vi "FieldInterference.vi"(0 "XCorner":dbl[](array[numeric]), 2 "Rotation":dbl, 5 "YCorner":dbl[](array[numeric]), 9 "Xsonde":dbl, 11 "Ysonde":dbl, 13 "Direction":dbl) -> (3 "vxx":dbl, 6 "XCible":dbl, 10 "YCible":dbl, 14 "vyy":dbl)   [LabVIEW 2011]
panel:
  out "D":bool
  out "C":bool
  out "A":bool
  out "B":bool
  out "d1y":dbl
  out "d1x":dbl
  out "c1y":dbl
  out "c1x":dbl
  out "b1y":dbl
  out "b1x":dbl
  out "output variable":dbl
  out "a1y":dbl
  out "a1x":dbl
  out "c2x":dbl
  out "c2y":dbl
  out "d2x":dbl
  out "d2y":dbl
  out "k1c":dbl
  out "k2c":dbl
  out "k1d":dbl
  out "k2d":dbl
  out "vDy":dbl
  out "vDx":dbl
  out "vCy":dbl
  out "vCx":dbl
  out "k2b":dbl
  out "k1b":dbl
  out "vBy":dbl
  out "vBx":dbl
  out "b2y":dbl
  out "b2x":dbl
  out "a2y":dbl
  out "a2x":dbl
  out "vAy":dbl
  out "vAx":dbl
  out "k2a":dbl
  out "k1a":dbl
  out "Theta":dbl
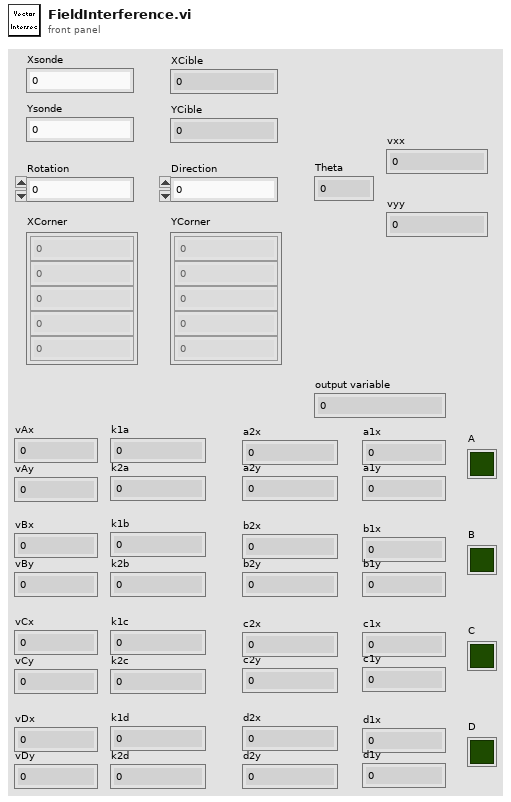
[diagram p1: front panel]
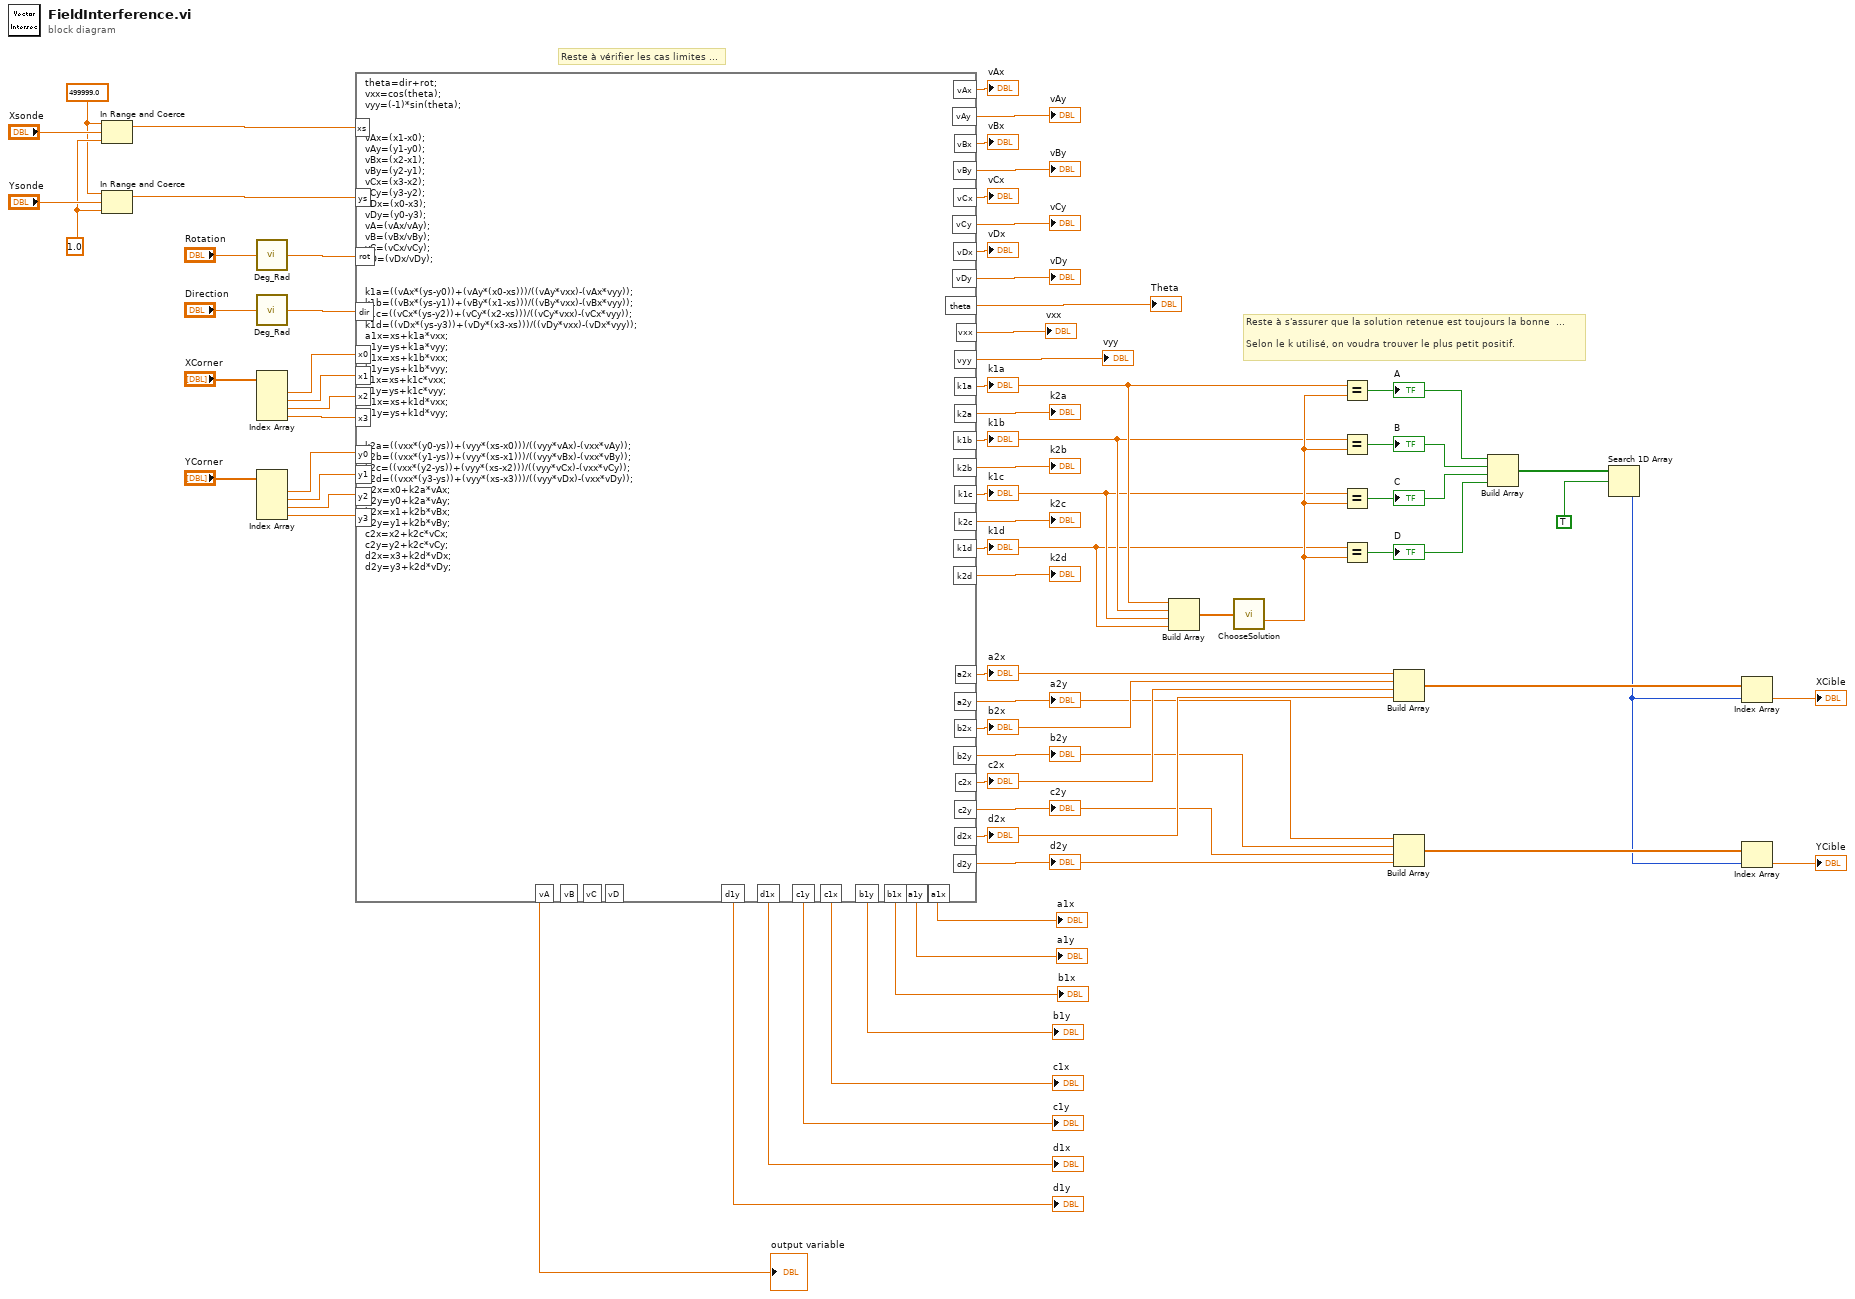
[diagram p0: block diagram]
diagram:
  w3 = 499999.0 ("upper limit")
  w4 = 1.0 ("lower limit")
  # "Reste à vérifier les cas limites ..."
  # "Reste à s'assurer que la solution retenue est toujours la bonne  ...\n\nSelon le k utilisé, on voudra trouver le plus petit positif."
  n1 = In Range and Coerce(upper limit=w3, x="Xsonde", lower limit=w4) -> (coerced(x)=w2:dbl)  [unwired: 1 out]
  n2 = In Range and Coerce(upper limit=w3, x="Ysonde", lower limit=w4) -> (coerced(x)=w1:dbl)  [unwired: 1 out]
  n3 = call "Deg_Rad.vi"("Angle"="Rotation") -> ("RadRot"=w58:dbl)
  n4 = call "Deg_Rad.vi"("Angle"="Direction") -> ("RadRot"=w56:dbl)
  n5 = Index Array(array="XCorner") -> (element #1=w68:dbl, element #2=w67:dbl, element #3=w66:dbl, element #4=w65:dbl)  [unwired: 4 in]
  n6 = Index Array(array="YCorner") -> (element #1=w64:dbl, element #2=w63:dbl, element #3=w62:dbl, element #4=w61:dbl)  [unwired: 4 in]
  n7 = formula code="theta=dir+rot;\nvxx=cos(theta);\nvyy=(-1)*sin(theta);\n\n\nvAx=(x1-x0);\nvAy=(y1-y0);\nvBx=(x2-x1);\nvBy=(y2-y1);\nvCx=(x3-x2);\nvCy=(y3-y2);\nvDx=(x0-x3);\nvDy=(y0-y3);\nvA=(vAx/vAy);\nvB=(vBx/vBy);\nvC=(vCx/vCy);\nvD=(vDx/vDy);\n\n\nk1a=((vAx*(ys-y0))+(vAy*(x0-xs)))/((vAy*vxx)-(vAx*vyy));\nk1b=((vBx*(ys-y1))+(vBy*(x1-xs)))/((vBy*vxx)-(vBx*vyy));\nk1c=((vCx*(ys-y2))+(vCy*(x2-xs)))/((vCy*vxx)-(vCx*vyy));\nk1d=((vDx*(ys-y3))+(vDy*(x3-xs)))/((vDy*vxx)-(vDx*vyy));\na1x=xs+k1a*vxx;\na1y=ys+k1a*vyy;\nb1x=xs+k1b*vxx;\nb1y=ys+k1b*vyy;\nc1x=xs+k1c*vxx;\nc1y=ys+k1c*vyy;\nd1x=xs+k1d*vxx;\nd1y=ys+k1d*vyy;\n\n\nk2a=((vxx*(y0-ys))+(vyy*(xs-x0)))/((vyy*vAx)-(vxx*vAy));\nk2b=((vxx*(y1-ys))+(vyy*(xs-x1)))/((vyy*vBx)-(vxx*vBy));\nk2c=((vxx*(y2-ys))+(vyy*(xs-x2)))/((vyy*vCx)-(vxx*vCy));\nk2d=((vxx*(y3-ys))+(vyy*(xs-x3)))/((vyy*vDx)-(vxx*vDy));\na2x=x0+k2a*vAx;\na2y=y0+k2a*vAy;\nb2x=x1+k2b*vBx;\nb2y=y1+k2b*vBy;\nc2x=x2+k2c*vCx;\nc2y=y2+k2c*vCy;\nd2x=x3+k2d*vDx;\nd2y=y3+k2d*vDy;"("x1"=w67, "x2"=w66, "x3"=w65, "x0"=w68, "y0"=w64, "y1"=w63, "y2"=w62, "y3"=w61, "rot"=w58, "xs"=w2, "ys"=w1, "dir"=w56) -> ("vAx"=→"vAx":dbl, "vAy"=→"vAy":dbl, "vBx"=→"vBx":dbl, "vBy"=→"vBy":dbl, "vCx"=→"vCx":dbl, "vCy"=→"vCy":dbl, "vDx"=→"vDx":dbl, "vDy"=→"vDy":dbl, "theta"=→"Theta":dbl, "vxx"=→"vxx":dbl, "vyy"=→"vyy":dbl, "k1a"=w29:dbl, "k2a"=→"k2a":dbl, "a2x"=w19:dbl, "a2y"=w12:dbl, "b2x"=w18:dbl, "b2y"=w13:dbl, "k2b"=→"k2b":dbl, "k1b"=w28:dbl, "k1c"=w27:dbl, "k2c"=→"k2c":dbl, "k1d"=w26:dbl, "k2d"=→"k2d":dbl, "c2x"=w17:dbl, "c2y"=w14:dbl, "d2x"=w16:dbl, "d2y"=w15:dbl, "vA"=→"output variable":dbl, "a1x"=→"a1x":dbl, "a1y"=→"a1y":dbl, "b1x"=→"b1x":dbl, "b1y"=→"b1y":dbl, "c1x"=→"c1x":dbl, "c1y"=→"c1y":dbl, "d1x"=→"d1x":dbl, "d1y"=→"d1y":dbl)  [unwired: 3 out]
  "k1a" <- w29
  "a2x" <- w19
  "a2y" <- w12
  "b2x" <- w18
  "b2y" <- w13
  "k1b" <- w28
  "k1c" <- w27
  "k1d" <- w26
  "c2x" <- w17
  "c2y" <- w14
  "d2x" <- w16
  "d2y" <- w15
  n8 = Build Array(w29, w28, w27, w26) -> (w31:dbl[])
  n9 = call "ChooseSolution.vi"("Solutions"=w31) -> ("min value"=w30:dbl)  [unwired: 14 in]
  n10 = Equal?(x=w29, y=w30) -> (x = y?=w22:bool)
  "A" <- w22
  n11 = Equal?(x=w28, y=w30) -> (x = y?=w23:bool)
  "B" <- w23
  n12 = Equal?(x=w27, y=w30) -> (x = y?=w24:bool)
  "C" <- w24
  n13 = Equal?(x=w26, y=w30) -> (x = y?=w25:bool)
  "D" <- w25
  n14 = Build Array(w19, w18, w17, w16) -> (w11:dbl[])
  n15 = Build Array(w12, w13, w14, w15) -> (w10:dbl[])
  n16 = Build Array(w22, w23, w24, w25) -> (w21:bool[])
  n17 = Search 1D Array(1D array=w21, element=TRUE) -> (index of element=w9:i32)  [unwired: 1 in]
  n18 = Index Array(array=w11, index=w9) -> (element=→"XCible":dbl)
  n19 = Index Array(array=w10, index=w9) -> (element=→"YCible":dbl)
